vi "types.create.vi"(8 "error in":errorcluster, 9 "Description":string, 10 "Name":string, 11 "Nominal Client in":refnum<class "Nominal Client.lvclass">) -> (0 "error out":errorcluster, 2 "type":refnum<class "type.lvclass">, 3 "Nominal Client out":refnum<class "Nominal Client.lvclass">)   [LabVIEW 2020, in "Nominal Client.lvclass"]
uses:
  Nominal Client.lvclass
  type/type.lvclass
  Nominal Client.lvclass/Nominal Client.ctl
  nominal types/workspace/workspace.lvclass/workspace.ctl
  4939f83f-28a0-422e-8382-4d9b1fcbd9ee.vi
  76140119-96e7-4153-8821-f12d461a7f7a.vi
  f0ddba77-c476-4c6f-9ef5-c6d42655afba.vi
  nominal types/workspace/rid.get.vi
  <vilib>/JDP Science/JSONtext/Variant to JSON Text.vi
  <vilib>/JDP Science/JSONtext/LVClass Serializer/JSONtext LVClass Serializer.lvclass
  <vilib>/JDP Science/JSONtext/JSONtext.lvlib
  nominal types/workspace/workspace.lvclass
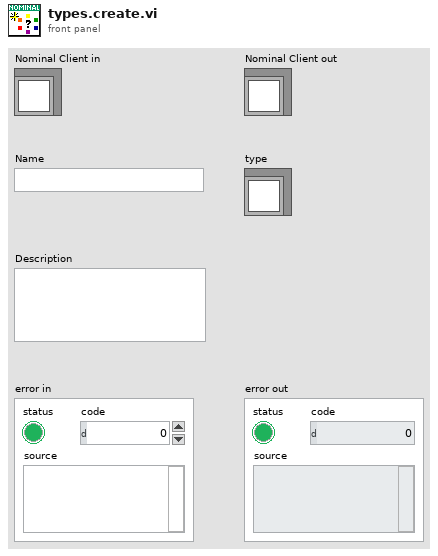
[diagram p1: front panel]
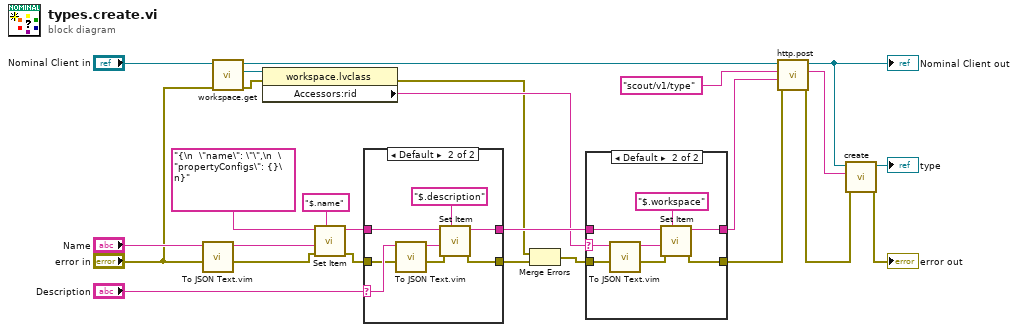
[diagram p0: block diagram]
diagram:
  n1 = call "To JSON Text.vim"("error in (no error)"="error in", "Anything"="Name") -> ("error out"=w19:errorcluster, "<JSON>"=w22:string)  [unwired: 8 in]
  n2 = call "workspace.get.vi"("error in"="error in", "Nominal Client in"="Nominal Client in") -> ("error out"=w14:errorcluster, "workspace"=w16:refnum<class "workspace.lvclass">, "Nominal Client out"=w9:refnum<class "Nominal Client.lvclass">)  [unwired: 7 in]
  n3 = property class="workspace.lvclass"(reference=w16, error in=w14) -> (error out=w11:errorcluster, "Accessors:rid"=w15:string)  [unwired: 1 out]
  n4 = call <vilib>:"Set Item.vi"("$Path or Item Name"="$.name", "error in (no error)"=w19, "JSON to Insert"=w22, "JSON"="{\n  \"name\": \"\",\n  \"propertyConfigs\": {}\n}") -> ("error out"=w20:errorcluster, "<JSON>"=w25:string)  [unwired: 4 in, 1 out]
  n5 = case shown="Default" "Description" {
    selector: "Description" -> [_ w34]
    tunnel: w25 -> [w28 w35]
    tunnel: [w28 w32] -> w18
    tunnel: w20 -> [w27 w31]
    tunnel: [w27 w29] -> w12
    frame "" {
    }
    frame Default {
      n6 = call "To JSON Text.vim"("error in (no error)"=w31, "Anything"=w34) -> ("error out"=w30:errorcluster, "<JSON>"=w33:string)  [unwired: 8 in]
      n7 = call <vilib>:"Set Item.vi"("$Path or Item Name"="$.description", "error in (no error)"=w30, "JSON to Insert"=w33, "JSON"=w35) -> ("error out"=w29:errorcluster, "<JSON>"=w32:string)  [unwired: 4 in, 1 out]
    }
  }
  n8 = Merge Errors(w11, w12) -> (w10:errorcluster)
  n9 = case shown="Default" w15 {
    selector: w15 -> [_ w44]
    tunnel: w18 -> [w38 w45]
    tunnel: [w38 w42] -> w8
    tunnel: w10 -> [w37 w39]
    tunnel: [w37 w40] -> w7
    frame "" {
    }
    frame Default {
      n10 = call "To JSON Text.vim"("error in (no error)"=w39, "Anything"=w44) -> ("error out"=w41:errorcluster, "<JSON>"=w43:string)  [unwired: 8 in]
      n11 = call <vilib>:"Set Item.vi"("$Path or Item Name"="$.workspace", "error in (no error)"=w41, "JSON to Insert"=w43, "JSON"=w45) -> ("error out"=w40:errorcluster, "<JSON>"=w42:string)  [unwired: 4 in, 1 out]
    }
  }
  n12 = call "http.post.vi"("error in"=w7, "Request body"=w8, "Path"="scout/v1/type", "Nominal Client in"=w9) -> ("error out"=w3:errorcluster, "Response"=w5:string, "Nominal Client out"=w4:refnum<class "Nominal Client.lvclass">)  [unwired: 5 in]
  "Nominal Client out" <- w4
  n13 = call "create.vi"("error in"=w3, "type"=w5, "Nominal Client"=w4) -> ("error out"=→"error out":errorcluster, "type"=→"type":refnum<class "type.lvclass">)  [unwired: 7 in]
